vi "Set Sequence Call Step Parameters.vi"(8 "error in (no error)":errorcluster, 11 "Generic DUT Setup in":refnum<class "Generic DUT Setup.lvclass">) -> (0 "error out":errorcluster, 3 "Generic DUT Setup out":refnum<class "Generic DUT Setup.lvclass">)   [LabVIEW 2016, in "Generic DUT Setup.lvlib" / "Generic DUT Setup.lvclass"]
uses:
  Generic DUT Setup.lvclass
  Plugins/String Database.lvlibp/String Database.lvclass
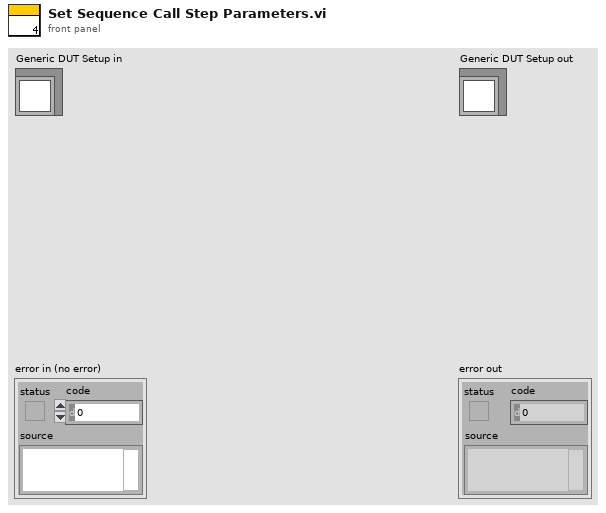
[diagram p1: front panel]
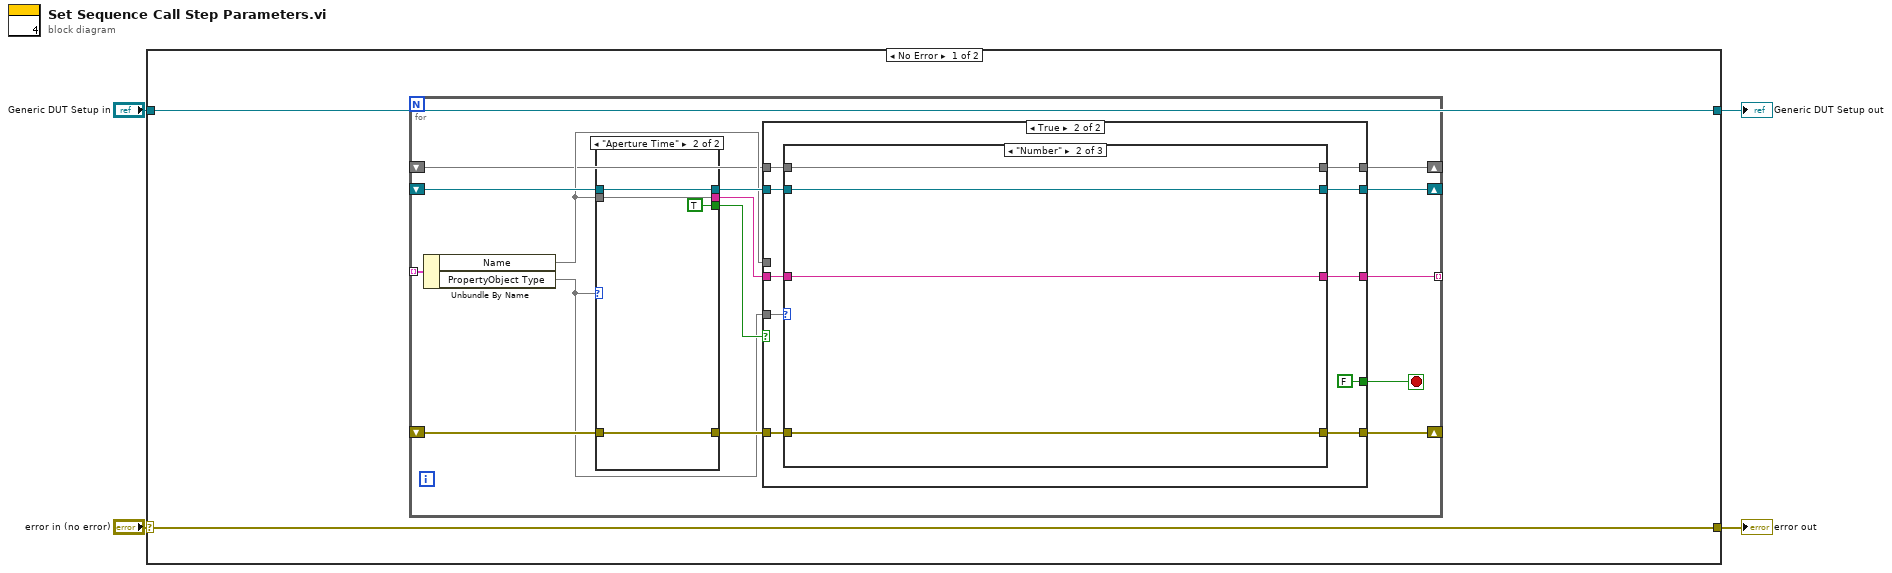
[diagram p0: block diagram]
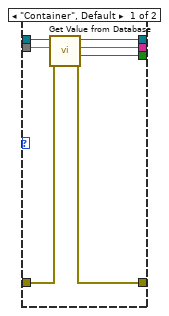
[diagram p2: hidden frame]
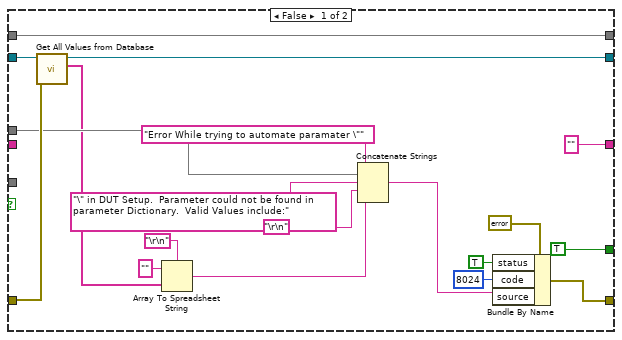
[diagram p3: hidden frame]
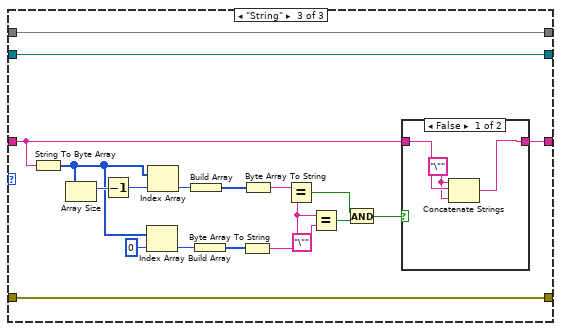
[diagram p5: hidden frame]
diagram:
  n1 = case shown="No Error" "error in (no error)" {
    selector: "error in (no error)" -> [w5 w94]
    tunnel: [w5 w94] -> w3
    tunnel: [w6 w93] -> w1
    tunnel: "Generic DUT Setup in" -> [w6 w93]
    frame No Error {
      n2 = for {
        tunnel: _ -> [w21] mode=indexing
        shift-right: [w15] -> _
        shift-left: _ -> [w20]
        shift-right: [w13] -> _
        shift-left: _ -> [w19]
        tunnel: [w16] -> _ mode=indexing
        shift-right: [w8] -> _
        shift-left: _ -> [w9]
        stop <- w11 stop-if-true
        n3 = Unbundle By Name(w21) -> ("Name"=w10, "PropertyObject Type"=w7)
        n4 = case shown="\"Aperture Time\"" w7 {
          tunnel: w20 -> [w28 w30]
          tunnel: w19 -> [w27 w32]
          tunnel: [w26 w31] -> w18
          tunnel: [w25 TRUE ("Entry Found")] -> w17
          tunnel: [w24 w30] -> w14
          tunnel: [w23 w32] -> w12
          tunnel: w10 -> [w22 w31]
          frame "Container", Default {
            n5 = call "Get Value from Database.vi"("error in (no error)"=w28, "Entry Name"=w22, "Message in"=w27) -> ("error out"=w24:errorcluster, "Entry Found"=w25:bool, "Entry Value"=w26:string, "Message out"=w23:refnum<class "String Database.lvclass">)  [unwired: 5 in]
          }
          frame "Aperture Time" {
          }
        }
        n6 = case shown="True" w17 {
          tunnel: w7 -> [_ w61]
          tunnel: w18 -> [_ w60]
          tunnel: ["" ("Entry Value") w59] -> w16
          tunnel: [w51 w56] -> w15
          tunnel: w14 -> [w41 w57]
          tunnel: [w42 w55] -> w13
          tunnel: w12 -> [w43 w54]
          tunnel: [TRUE ("status") FALSE ("status")] -> w11
          tunnel: w10 -> [w35 _]
          tunnel: w9 -> [w33 w53]
          tunnel: [w33 w52] -> w8
          frame False {
            n7 = call "Get All Values from Database.vi"("error in (no error)"=w41, "String Database in"=w43) -> ("Names"=w34:string[], "String Database out"=w42:refnum<class "String Database.lvclass">)  [unwired: 6 in, 2 out]
            n8 = Array To Spreadsheet String(delimiter (Tab)="\r\n", array=w34, 3:"" ("format string")) -> (spreadsheet string=w38:string)
            n9 = Concatenate Strings("Error While trying to automate paramater \"", w35, "\" in DUT Setup.  Parameter could not be found in parameter Dictionary.  Valid Values include:" ("string"), "\r\n", w38) -> (w45:string)
            n10 = Bundle By Name(cluster=errorcluster {"status"=FALSE, "code"=0, "source"=""} ("error out"), "status"=TRUE, "code"=8024, "source"=w45) -> (w51:errorcluster)
          }
          frame True {
            n11 = case shown="\"Number\"" w61 {
              tunnel: w60 -> [w65 w69 w73]
              tunnel: [w65 w69 w74] -> w59
              tunnel: w57 -> [w64 w68 w72]
              tunnel: [w64 w68 w72] -> w56
              tunnel: [w63 w67 w71] -> w55
              tunnel: w54 -> [w63 w67 w71]
              tunnel: w53 -> [w62 w66 w70]
              tunnel: [w62 w66 w70] -> w52
              frame "Container", Default {
              }
              frame "Number" {
              }
              frame "String" {
                n12 = String To Byte Array(string=w73) -> (unsigned byte array=w86:u8[])
                n13 = Array Size(array=w86) -> (size(s)=w88:i32)
                n14 = Decrement(x=w88) -> (x-1=w87:i32)
                n15 = Index Array(array=w86, index=0) -> (element=w84:u8)
                n16 = Index Array(array=w86, index=w87) -> (element=w85:u8)
                n17 = Build Array(w85) -> (w82:u8[])
                n18 = Build Array(w84) -> (w83:u8[])
                n19 = Byte Array To String(unsigned byte array=w83) -> (string=w80:string)
                n20 = Byte Array To String(unsigned byte array=w82) -> (string=w81:string)
                n21 = Equal?(x=w81, y=w80) -> (x = y?=w77:bool)
                n22 = Equal?(x=w80, y="\"") -> (x = y?=w78:bool)
                n23 = And(x=w77, y=w78) -> (x .and. y?=w75:bool)
                n24 = case shown="False" w75 {
                  tunnel: [w90 w92] -> w74
                  tunnel: w73 -> [w91 w92]
                  frame False {
                    w89 = "\"" ("string")
                    n25 = Concatenate Strings(w89, w91, w89) -> (w90:string)
                  }
                  frame True {
                  }
                }
              }
            }
          }
        }
      }
    }
    frame Error {
    }
  }
  "error out" <- w3
  "Generic DUT Setup out" <- w1
